vi "tra25cc_goto_xy-absolute.vi"(8 "error in (no error)":errorcluster, 10 "xy_val_mm":cluster{"x_val":dbl, "y_val":dbl}, 11 "conn_xyz_in":T2) -> (0 "error out":errorcluster, 3 "conn_xyz_out":T1)   [LabVIEW 2018]
uses:
  D:/Data/Thea/tests/Labview/Scanner_v3_Phy-2019.05.06/src/Stage_xyz/Dll/Newport.CONEXCC.CommandInterface.dll
  Dll/Newport.CONEXCC.CommandInterface.dll
  GLOBAL_VAR.vi
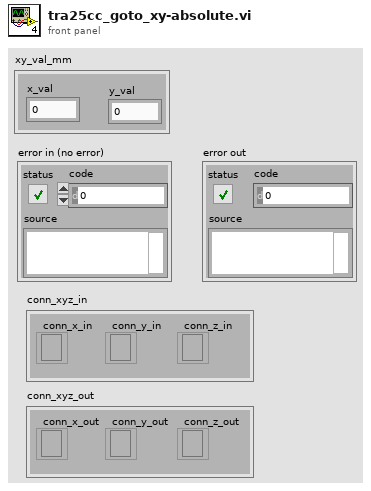
[diagram p1: front panel]
types:
  T1 = cluster{"conn_x_out":refnum<k24>, "conn_y_out":refnum<k24>, "conn_z_out":refnum<k24>}
  T2 = cluster{"conn_x_in":refnum<k24>, "conn_y_in":refnum<k24>, "conn_z_in":refnum<k24>}
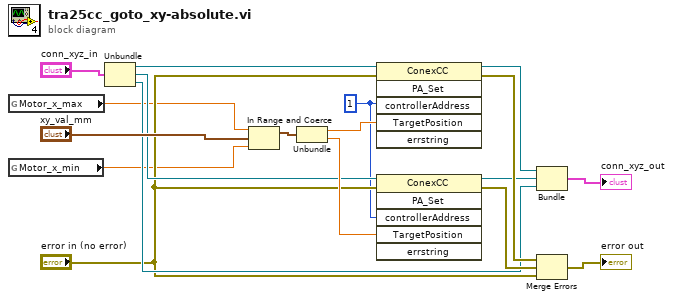
[diagram p0: block diagram]
diagram:
  w3 = 1 ("controllerAddress")
  n1 = global read "GLOBAL_VAR.vi" "Motor_x_max"() -> (w2:dbl)
  n2 = global read "GLOBAL_VAR.vi" "Motor_x_min"() -> (w1:dbl)
  n3 = Unbundle("conn_xyz_in") -> ("conn_x_in"=w7:refnum<k24>, "conn_y_in"=w6:refnum<k24>, "conn_z_in"=w5:refnum<k24>)
  n4 = In Range and Coerce(upper limit=w2, x="xy_val_mm", lower limit=w1) -> (coerced(x)=w8:cluster{"x_val":dbl, "y_val":dbl})  [unwired: 1 out]
  n5 = Unbundle(w8) -> ("x_val"=w14:dbl, "y_val"=w13:dbl)
  n6 = invoke class="ConexCC" method="PA_Set"(reference=w7, error in="error in (no error)", "controllerAddress"=w3, "TargetPosition"=w14) -> (reference out=w11:refnum<k24>, error out=w16:errorcluster)  [unwired: 2 in, 4 out]
  n7 = invoke class="ConexCC" method="PA_Set"(reference=w6, error in="error in (no error)", "controllerAddress"=w3, "TargetPosition"=w13) -> (reference out=w10:refnum<k24>, error out=w17:errorcluster)  [unwired: 2 in, 4 out]
  n8 = Bundle("conn_x_in"=w11, "conn_y_in"=w10, "conn_z_in"=w5) -> (→"conn_xyz_out":T2)  [unwired: 1 in]
  n9 = Merge Errors(w16, w17, "error in (no error)") -> (→"error out":errorcluster)
